vi "Create Extended Messages.vi"() -> ()   [LabVIEW 2011]
uses:
  Program Files/National Instruments/LabVIEW 2011/examples/nixnet/examples.llb/NI-XNET Example Control - CAN Frame.ctl
  Program Files/National Instruments/LabVIEW 2011/examples/nixnet/examples.llb/NI-XNET Example Control - Signal.ctl
  Program Files/National Instruments/LabVIEW 2011/resource/objmgr/xnet.rc
panel:
  out "error out":errorcluster
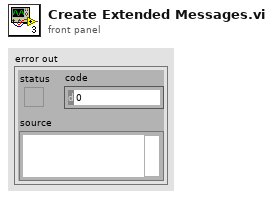
[diagram p1: front panel]
types:
  T1 = typedef "NI-XNET Example Control - CAN Frame.ctl" = cluster{"Frame name":string, "Identifier":u32, "Payload Length":u32, "Timing Type":u32, "Transmit Time":dbl, "Extended Identifier?":bool, "Comment":string}
  T2 = typedef "NI-XNET Example Control - Signal.ctl" = cluster{"Signal name":string, "Scaling Factor":dbl, "Scaling Offset":dbl, "Maximum Value":dbl, "Minimum Value":dbl, "Default Value":dbl, "Unit":string, "Start Bit":u32, "Number of Bits":u32, "Data Type":u32, "Byte Order":u32, "Comment":string}
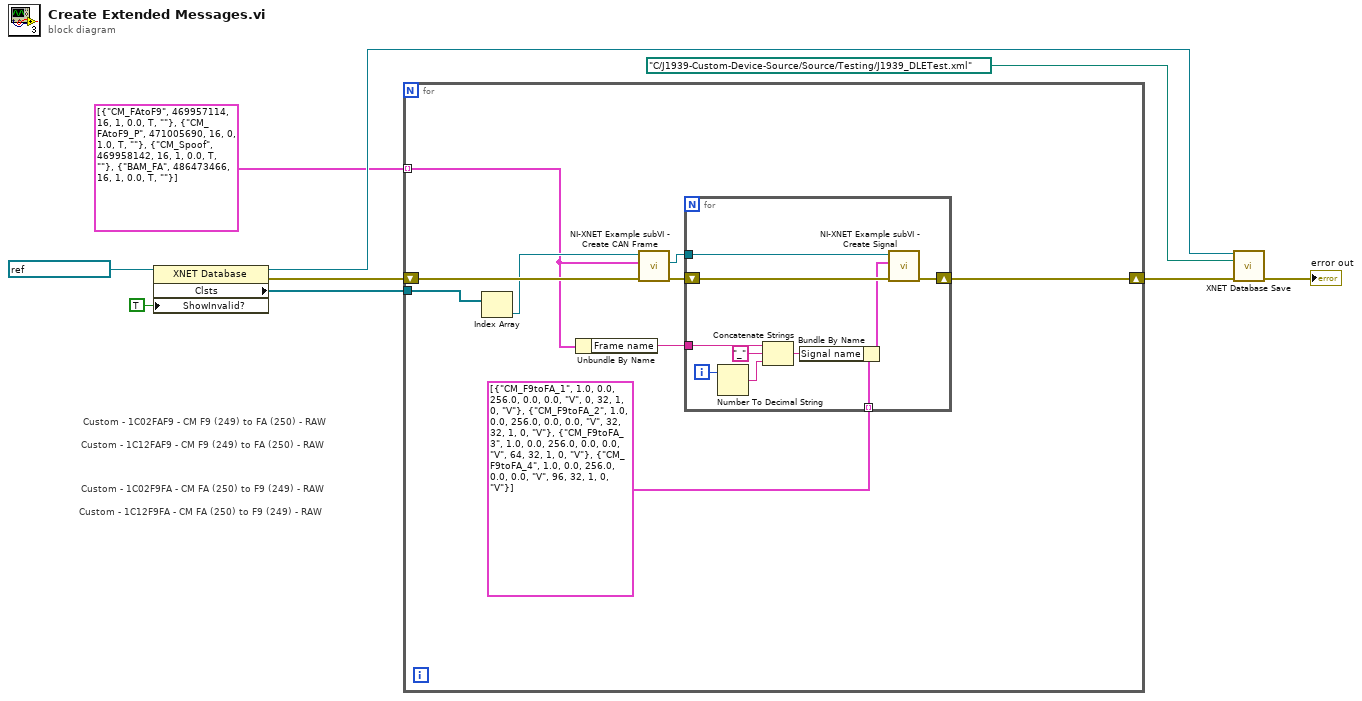
[diagram p0: block diagram]
diagram:
  # "Custom - 1C12F9FA - CM FA (250) to F9 (249) - RAW"
  # "Custom - 1C12FAF9 - CM F9 (249) to FA (250) - RAW"
  # "Custom - 1C02F9FA - CM FA (250) to F9 (249) - RAW"
  # "Custom - 1C02FAF9 - CM F9 (249) to FA (250) - RAW"
  n1 = property class="XNET Database"(reference=refnum<k21> "J1939_DLETest" ("XNET Database"), "ShowInvalid?"=TRUE ("Show Invalid From Open?")) -> (reference out=w3:refnum<k21>, error out=w7:errorcluster, "Clsts"=w8:refnum<k21>[])  [unwired: 1 in]
  n2 = for {
    tunnel: w8 -> [w18]
    tunnel: T1[] [{"Frame name"="CM_FAtoF9", "Identifier"=469957114, "Payload Length"=16, "Timing Type"=1, "Transmit Time"=0.0, "Extended Identifier?"=TRUE, "Comment"=""}, {"Frame name"="CM_FAtoF9_P", "Identifier"=471005690, "Payload Length"=16, "Timing Type"=0, "Transmit Time"=1.0, "Extended Identifier?"=TRUE, "Comment"=""}, {"Frame name"="CM_Spoof", "Identifier"=469958142, "Payload Length"=16, "Timing Type"=1, "Transmit Time"=0.0, "Extended Identifier?"=TRUE, "Comment"=""}, {"Frame name"="BAM_FA", "Identifier"=486473466, "Payload Length"=16, "Timing Type"=1, "Transmit Time"=0.0, "Extended Identifier?"=TRUE, "Comment"=""}] -> [w11] mode=indexing
    shift-right: [w12] -> w5
    shift-left: w7 -> [w17]
    n3 = Index Array(array=w18) -> (element=w16:refnum<k21>)  [unwired: 1 in]
    n4 = Unbundle By Name(w11) -> ("Frame name"=w10:string)
    n5 = call "NI-XNET Example subVI - Create CAN Frame.vi"("error in"=w17, "CAN Frame"=w11, "cluster in"=w16) -> ("error out"=w15:errorcluster, "frame out"=w14:refnum<k21>)  [unwired: 3 in, 4 out]
    n6 = for {
      tunnel: w14 -> [w27]
      shift-right: [w26] -> w12
      shift-left: w15 -> [w28]
      tunnel: T2[] [{"Signal name"="CM_F9toFA_1", "Scaling Factor"=1.0, "Scaling Offset"=0.0, "Maximum Value"=256.0, "Minimum Value"=0.0, "Default Value"=0.0, "Unit"="V", "Start Bit"=0, "Number of Bits"=32, "Data Type"=1, "Byte Order"=0, "Comment"="V"}, {"Signal name"="CM_F9toFA_2", "Scaling Factor"=1.0, "Scaling Offset"=0.0, "Maximum Value"=256.0, "Minimum Value"=0.0, "Default Value"=0.0, "Unit"="V", "Start Bit"=32, "Number of Bits"=32, "Data Type"=1, "Byte Order"=0, "Comment"="V"}, {"Signal name"="CM_F9toFA_3", "Scaling Factor"=1.0, "Scaling Offset"=0.0, "Maximum Value"=256.0, "Minimum Value"=0.0, "Default Value"=0.0, "Unit"="V", "Start Bit"=64, "Number of Bits"=32, "Data Type"=1, "Byte Order"=0, "Comment"="V"}, {"Signal name"="CM_F9toFA_4", "Scaling Factor"=1.0, "Scaling Offset"=0.0, "Maximum Value"=256.0, "Minimum Value"=0.0, "Default Value"=0.0, "Unit"="V", "Start Bit"=96, "Number of Bits"=32, "Data Type"=1, "Byte Order"=0, "Comment"="V"}] -> [w22] mode=indexing
      tunnel: w10 -> [w24]
      i -> [w25]
      n7 = Number To Decimal String(number=w25) -> (decimal integer string=w23:string)  [unwired: 1 in]
      n8 = Concatenate Strings(w24, "_" ("string"), w23) -> (w21:string)
      n9 = Bundle By Name(cluster=w22, "Signal name"=w21) -> (w19:T2)
      n10 = call "NI-XNET Example subVI - Create Signal.vi"("error in"=w28, "Signal Cluster"=w19, "frame in"=w27) -> ("error out"=w26:errorcluster)  [unwired: 8 out]
    }
  }
  n11 = call <vilib>:"XNET Database Save.vi"("database in"=w3, "filepath (empty)"=path "C:/J1939-Custom-Device-Source/Source/Testing/J1939_DLETest.xml", "error in (no error)"=w5) -> ("error out"=→"error out":errorcluster)  [unwired: 11 in, 1 out]
